vi "Get Error.vi"(11 "TEMPLATE jettl in":refnum<class "TEMPLATE Actor.lvclass">) -> (2 "Error":errorcluster)   [LabVIEW 2021, in "_Template.lvlib" / "Templates.lvlib" / "TEMPLATE Actor.lvlib" / "TEMPLATE Actor.lvclass"]
uses:
  TEMPLATE Actor.lvclass
  jettl/jettl/jettl/jettl.lvclass
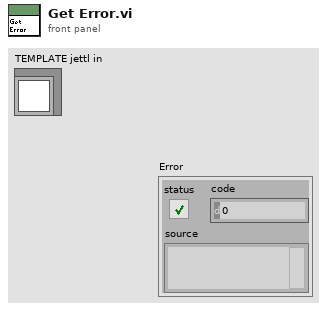
[diagram p1: front panel]
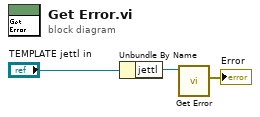
[diagram p0: block diagram]
diagram:
  n1 = Unbundle By Name("TEMPLATE jettl in") -> ("jettl"=w2:refnum<class "jettl.lvclass">)
  n2 = call-dynamic "Get Error.vi"("jettl in"=w2) -> ("Error"=→"Error":errorcluster)  [unwired: 10 in]
